vi "temperature gauge.vi"() -> ()   [LabVIEW 2018]
panel:
  in  "delay":string
  in  "stop":bool
  in  "Celcius?":bool=TRUE
  in  "Temperature":dbl(slide) scale=0.0..100.0
  out "Fahrenheit":dbl
  out "Celcius":dbl
  out "Thermometer":dbl(slide) scale=0.0..100.0
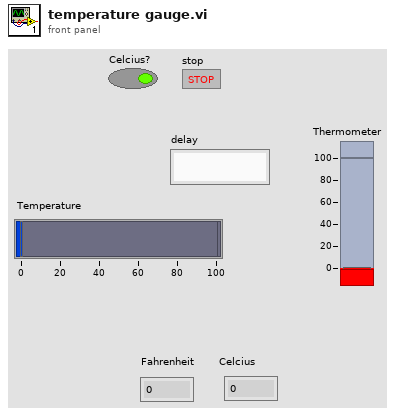
[diagram p1: front panel]
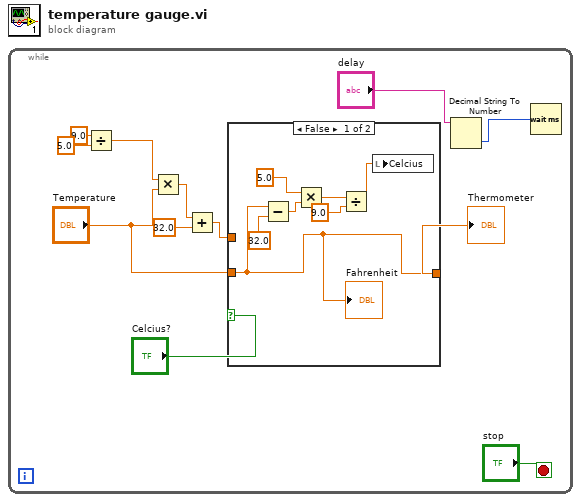
[diagram p0: block diagram]
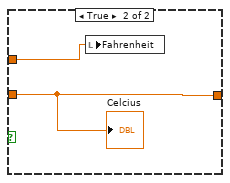
[diagram p2: hidden frame]
diagram:
  n1 = while {
    stop <- "stop" stop-if-true
    n2 = Divide(x=9.0, y=5.0) -> (x/y=w5:dbl)
    n3 = Multiply(x=w5, y="Temperature") -> (x*y=w9:dbl)
    n4 = Add(x=w9, y=32.0) -> (x+y=w7:dbl)
    n5 = case shown="False" "Celcius?" {
      tunnel: w7 -> [_ w20]
      tunnel: [w15 w21] -> w3
      tunnel: "Temperature" -> [w15 w21]
      frame False {
        n6 = Subtract(x=w15, y=32.0 ("x")) -> (x-y=w19:dbl)
        n7 = Multiply(x=5.0, y=w19) -> (x*y=w13:dbl)
        n8 = Divide(x=w13, y=9.0 ("x")) -> (x/y=w18:dbl)
        n9 = local write "Celcius"(w18) -> ()
        "Fahrenheit" <- w15
      }
      frame True {
        n10 = local write "Fahrenheit"(w20) -> ()
        "Celcius" <- w21
      }
    }
    "Thermometer" <- w3
    n11 = Decimal String To Number(string="delay") -> (number=w2:i32)  [unwired: 2 in, 1 out]
    n12 = Wait (ms)(milliseconds to wait=w2) -> ()  [unwired: 1 out]
  }
